vi "gainSnake.vi"(8 "error in (no error)":errorcluster, 11 "Snake in":refnum<class "Snake.lvclass">) -> (0 "error out":errorcluster, 3 "Snake out":refnum<class "Snake.lvclass">)   [LabVIEW 2014, in "Snake.lvclass"]
uses:
  Snake.lvclass
  Snake.lvclass/Snake.ctl
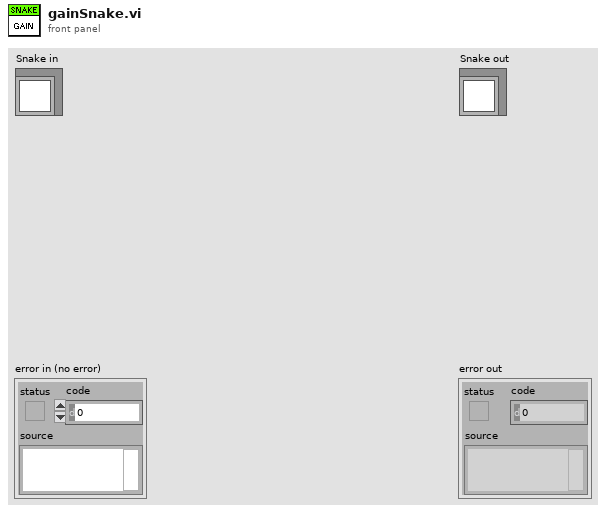
[diagram p1: front panel]
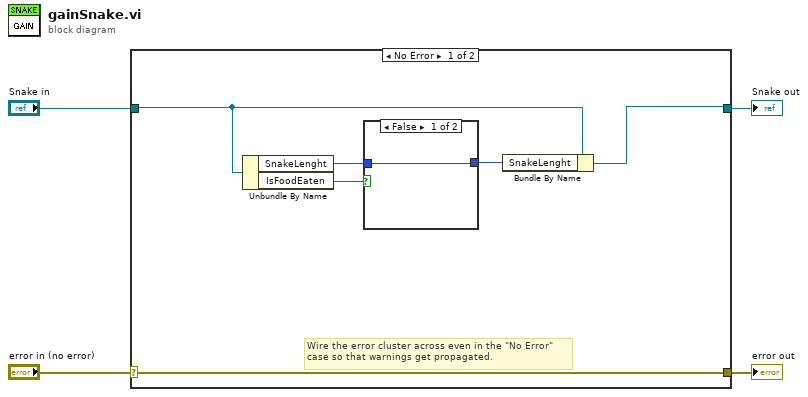
[diagram p0: block diagram]
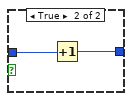
[diagram p2: hidden frame]
diagram:
  n1 = case shown="No Error" "error in (no error)" {
    selector: "error in (no error)" -> [w10 w15]
    tunnel: [w10 w15] -> w3
    tunnel: [w6 w14] -> w1
    tunnel: "Snake in" -> [w8 w14]
    frame No Error {
      # "Wire the error cluster across even in the \"No Error\"\ncase so that warnings get propagated."
      n2 = Unbundle By Name(w8) -> ("SnakeLenght"=w9:u32, "IsFoodEaten"=w5:bool)
      n3 = case shown="False" w5 {
        tunnel: w9 -> [w11 w13]
        tunnel: [w11 w12] -> w7
        frame False {
        }
        frame True {
          n4 = Increment(x=w13) -> (x+1=w12:u32)
        }
      }
      n5 = Bundle By Name(cluster=w8, "SnakeLenght"=w7) -> (w6:refnum<class "Snake.lvclass">)
    }
    frame Error {
    }
  }
  "error out" <- w3
  "Snake out" <- w1
